vi "NI.StatechartInstantiateVI 4.vi"(3 "State/Inputs/Outputs in":T1) -> (0 "Execute?":bool)   [LabVIEW 2013]
uses:
  iRobot Navigation State Machine.lvsc/GencodeCluster.ctl
  iRobot Navigation State Machine.lvsc
panel:
  in  "Execute Ctl":cluster{"Execute?":bool}
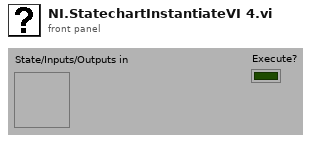
[diagram p1: front panel]
types:
  T1 = typedef "iRobot Navigation State Machine.lvsc/GencodeCluster.ctl" = cluster{"RW":cluster{"Outputs":T2, "StateData":T3, "InternalQueue":T4}, "R":cluster{"Inputs":T6, "StatechartState":T16}}
  T2 = typedef "iRobot Navigation State Machine.lvsc/Outputs.ctl" = cluster{"Left Wheel Speed (mm/s)":i16, "Right Wheel Speed (mm/s)":i16}
  T3 = typedef "iRobot Navigation State Machine.lvsc/StateData.ctl" = cluster{"distance at maneuver start (mm)":i32, "angle at maneuver start (deg)":i32}
  T4 = typedef "iRobot Navigation State Machine.lvsc/InternalQueue.ctl" = cluster{"Data":T5[], "Next Slot":u32, "Current Slot":u32, "Size":u32}
  T5 = typedef "iRobot Navigation State Machine.lvsc/Trigger.ctl" = enum16{"NULL"}
  T6 = typedef "iRobot Navigation State Machine.lvsc/Inputs.ctl" = cluster{"net distance (mm)":i32, "net angle (deg)":i32, "Max Wheel Speed (mm/s)":i16, "accelerometer":T7, "iRobot Sensors":T8, "Is Simulator?":bool, "Green":bool, "Red":bool}
  T7 = typedef "Accelerometer.ctl" = cluster{"x axis (g)":dbl, "y axis (g)":dbl, "z axis (g)":dbl}
  T8 = typedef "Sensor Group 6.ctl" = cluster{"Bumps + Wheel Drops":T9, "Wall":bool, "Cliff Left":bool, "Cliff Front Left":bool, "Cliff Front Right":bool, "Cliff Right":bool, "Virtual Wall":bool, "Low-Side Driver + Wheel Overcurrent":T10, "Infrared":u8, "Buttons":T11, "Distance (mm)":i32, "Angle (deg)":i32, "Charging State":T12, "Voltage (mV)":u16, "Current (mA)":i16, "Battery Temperature (deg C)":i8, "Battery Charge (mAh)":u16, "Battery Capacity (mAh)":u16, "Wall Signal (0-4095)":u16, "Cliff Left Signal (0-4095)":u16, "Cliff Front Left Signal (0-4095)":u16, "Cliff Front Right Signal (0-4095)":u16, "Cliff Right Signal (0-4095)":u16, "Cargo Bay Digital Inputs":T13, "Cargo Bay Analog Signal (0-1023)":u16, "Charging Sources Available":T14, "OI Mode":T15, "Song Number":u8, "Song Playing":bool, "Number of Stream Packets":u8, "Requested Velocity (mm/s)":i16, "Requested Radius (mm)":i16, "Requested Right Wheel Velocity (mm/s)":i16, "Requested Left Wheel Velocity (mm/s)":i16}
  T9 = typedef "Bumps + Wheel Drops.ctl" = cluster{"Wheeldrop Caster":bool, "Wheeldrop Left":bool, "Wheeldrop Right":bool, "Bump Left":bool, "Bump Right":bool}
  T10 = typedef "Low-Side Driver + Wheel Overcurrent.ctl" = cluster{"Low-Side Driver 0":bool, "Low-Side Driver 1":bool, "Low-Side Driver 2":bool, "Left Wheel":bool, "Right Wheel":bool}
  T11 = typedef "Buttons.ctl" = cluster{"Advance":bool, "Play":bool}
  T12 = typedef "Charging State.ctl" = enum16{"Not Charging", "Reconditioning Charging", "Full Charging", "Trickle Charging", "Waiting", "Charging Fault Condition"}
  T13 = typedef "Cargo Bay Digital Inputs.ctl" = cluster{"Digital Input 0":bool, "Digital Input 1":bool, "Digital Input 2":bool, "Digital Input 3":bool, "Device Detect":bool}
  T14 = typedef "Charging Sources Available.ctl" = cluster{"Internal Charger":bool, "Home Base":bool}
  T15 = typedef "OI Mode.ctl" = enum16{"Off", "Passive", "Safe", "Full"}
  T16 = typedef "iRobot Navigation State Machine.lvsc/StatechartState.ctl" = T17[]
  T17 = typedef "iRobot Navigation State Machine.lvsc/State.ctl" = enum16{"NI.SC.Initial", "NI.SC.History", "NI.SC.ShallowHistory", "NI.SC.Terminal", "Pause", "Run", "Pause\\Detect Play Button\\Pause;\nWait for\nbutton\nrelease", "Pause\\Detect Play Button\\Unpause;\nwait for\nbutton release", "Pause\\Detect Play Button\\Unpause;\nwait for\nbutton press", "Run\\Detect Obstacles\\NI.SC.UnnamedState 0", "Run\\Detect Obstacles\\Hit right side", "Run\\Detect Obstacles\\Hit left side", "Run\\Detect Obstacles\\Front Crossing the Line", "Run\\Detect Obstacles\\Right Passing", "Run\\Detect Obstacles\\Left Passing", "Run\\Detect Obstacles\\Hit the line", "Run\\Detect Obstacles\\Drive"}
  T18 = cluster{"Outputs":T2, "StateData":T3, "InternalQueue":T4}
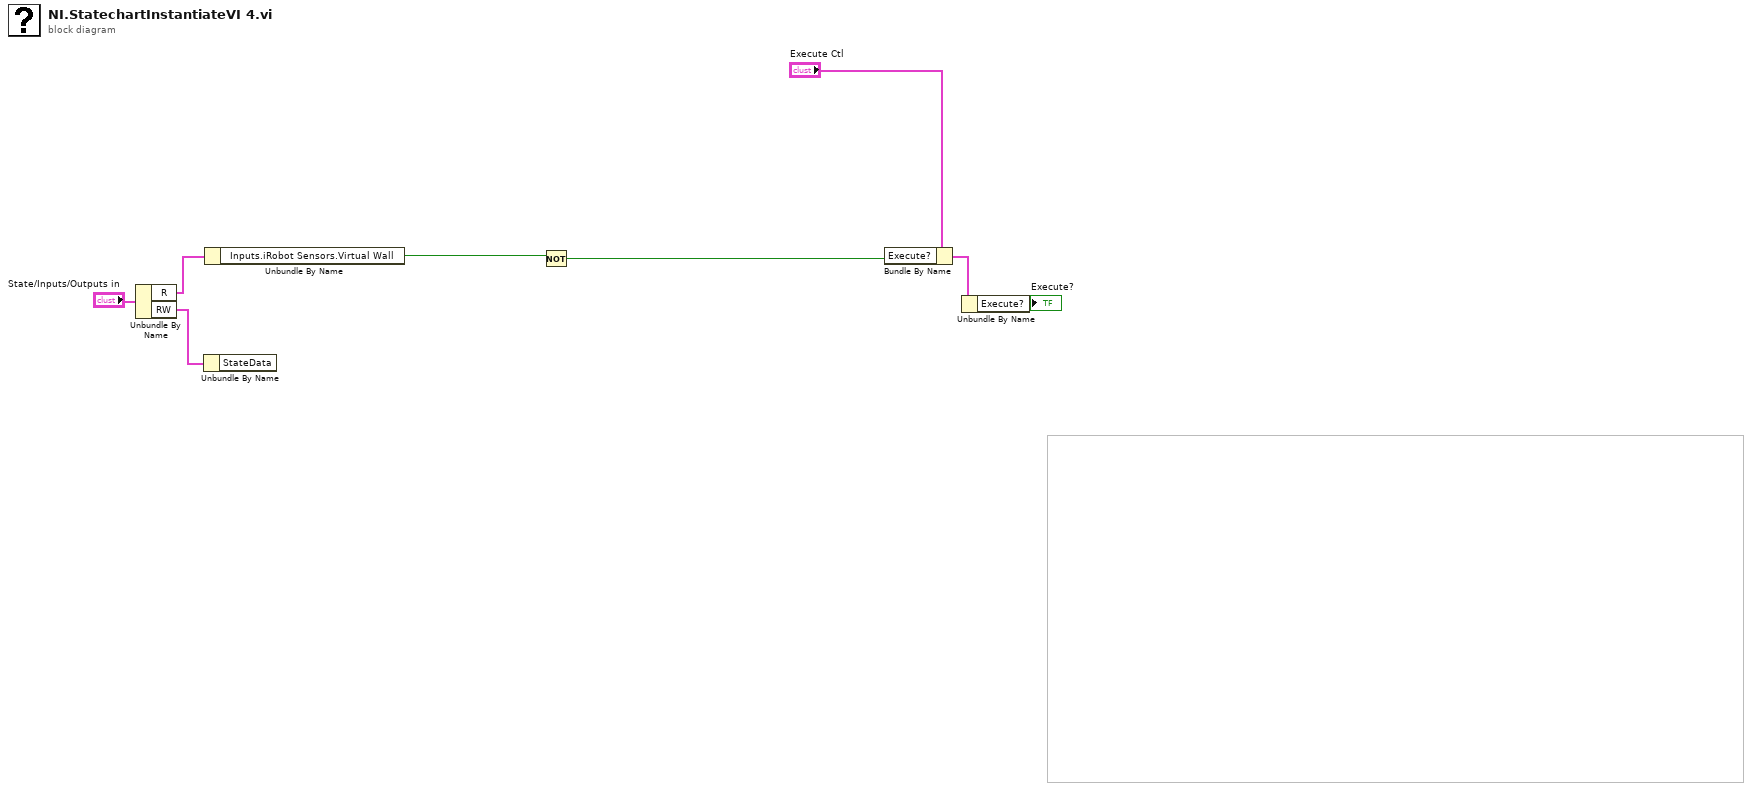
[diagram p0: block diagram]
diagram:
  n1 = Unbundle By Name("State/Inputs/Outputs in") -> ("R"=w3:cluster{"Inputs":T6, "StatechartState":T16}, "RW"=w4:T18)
  n2 = Unbundle By Name ("SCInRWSocket")(w4) -> ()  [unwired: 1 out]
  n3 = Unbundle By Name ("SCInRSocket")(w3) -> ("Inputs.iRobot Sensors.Virtual Wall"=w2:bool)
  n4 = Not(x=w2) -> (.not. x?=w1:bool)
  n5 = Bundle By Name ("SCOutSocket")(cluster="Execute Ctl", "Execute?"=w1) -> (w7:cluster{"Execute?":bool})
  n6 = Unbundle By Name(w7) -> ("Execute?"=→"Execute?":bool)
